vi "Drive Ref.vi"(5 "Wait for Completion (F)":bool, 6 "Timeout ms (-1)":i32, 7 "Locking? (F)":bool, 8 "error in":errorcluster, 9 "Force? (F)":bool, 10 "Data":variant, 11 "VI Refnum":refnum<vi>) -> (0 "error out":errorcluster, 3 "Queued Msg":T1)   [LabVIEW 2016, in "Drive System.lvlib"]
uses:
  Drive System.lvlib
  DriveCmd.ctl
  DriveCmdList.ctl
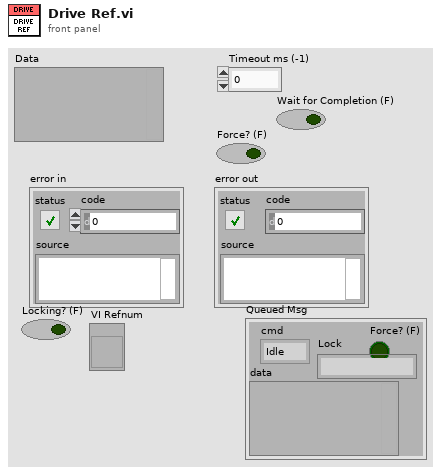
[diagram p1: front panel]
types:
  T1 = typedef "Drive System.lvlib/DriveCmd.ctl" = cluster{"cmd":T2, "data":variant, "Force? (F)":bool, "Lock":string}
  T2 = typedef "Drive System.lvlib/DriveCmdList.ctl" = enum16{"Idle", "Cleanup", "Drive For Time", "Follow Path Speed Control", "Follow Path", "Drive Tank", "Drive Angle Mag", "Drive Arcade", "Drive Ref", "Unlock", "Lock"}
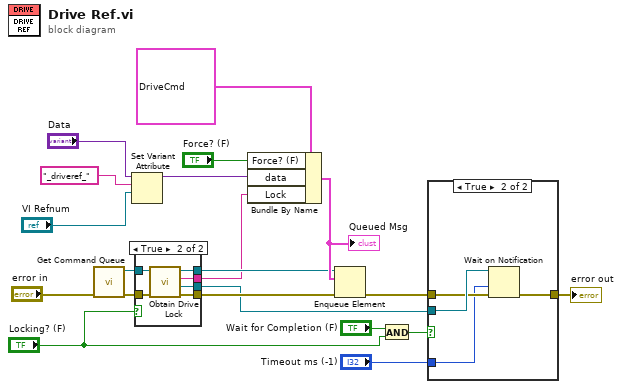
[diagram p0: block diagram]
diagram:
  n1 = call "Get Command Queue.vi"("error in (no error)"="error in") -> ("error out"=w19:errorcluster, "Queue out"=w11:refnum<queue>)  [unwired: 9 in]
  n2 = Set Variant Attribute(Variant="Data", name="_driveref_", value="VI Refnum") -> (Variant out=w13:variant)  [unwired: 1 in, 2 out]
  n3 = case shown="True" "Locking? (F)" {
    tunnel: w19 -> [w21 w28]
    tunnel: [w21 w27] -> w12
    tunnel: w11 -> [w22 w26]
    tunnel: [w22 w25] -> w10
    tunnel: [_ w24] -> w9
    tunnel: [_ w23] -> w6
    frame False {
    }
    frame True {
      n4 = call "Obtain Drive Lock.vi"("error in"=w28, "Queue in"=w26) -> ("error out"=w27:errorcluster, "notifier out"=w23:refnum<notifier>, "Lock"=w24:string, "queue out"=w25:refnum<queue>)  [unwired: 6 in]
    }
  }
  n5 = Bundle By Name(cluster=T1 {"cmd"=enum."Drive Ref", "data"=variant, "Force? (F)"=FALSE, "Lock"=""} ("element"), "Force? (F)"="Force? (F)", "data"=w13, "Lock"=w9) -> (w16:T1)
  "Queued Msg" <- w16
  n6 = Enqueue Element(queue=w10, element=w16, error in (no error)=w12) -> (error out=w7:errorcluster)  [unwired: 1 in, 2 out]
  n7 = And(x="Wait for Completion (F)", y="Locking? (F)") -> (x .and. y?=w3:bool)
  n8 = case shown="True" w3 {
    tunnel: w7 -> [w29 w32]
    tunnel: w6 -> [_ w33]
    tunnel: [w29 w31] -> w8
    tunnel: "Timeout ms (-1)" -> [_ w30]
    frame False {
    }
    frame True {
      n9 = Wait on Notification(notifier=w33, timeout in ms (-1)=w30, error in (no error)=w32) -> (error out=w31:errorcluster)  [unwired: 1 in, 3 out]
    }
  }
  "error out" <- w8
